vi "SmartSEM Remote API FIB mode.vi"(5 "Wait (ms)":u32, 7 "Iterations":u32=3, 8 "error in":errorcluster, 10 "FIB mode":T1(ring), 11 "ActiveX Container":refnum<k7>(container)) -> (0 "error out":errorcluster, 3 "reference out":refnum<k7>)   [LabVIEW 2018]
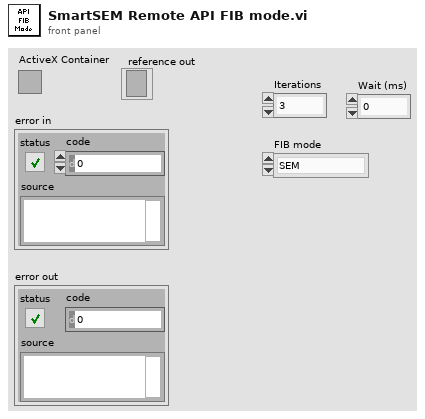
[diagram p1: front panel]
types:
  T1 = enum16{"SEM", "FIB", "Mill", "SEM + FIB", "Mill + SEM", "Drift SEM", "Drift FIB", "None", "Ext", "Ext + SEM"}
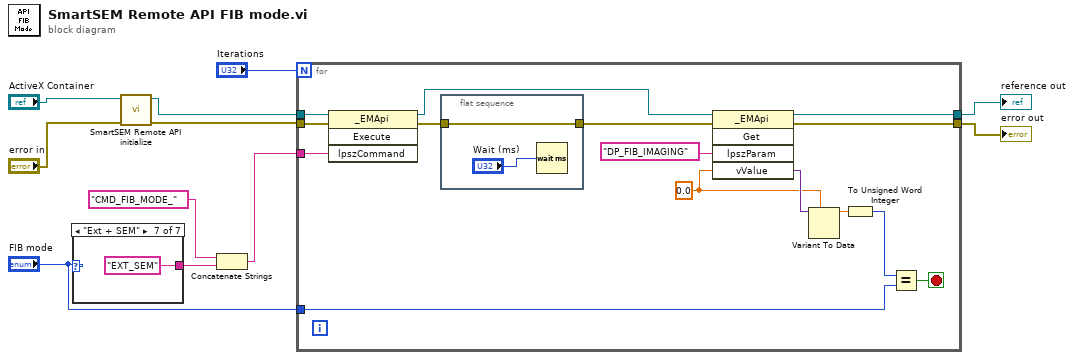
[diagram p0: block diagram]
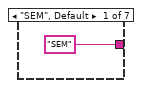
[diagram p2: hidden frame]
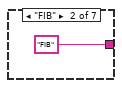
[diagram p3: hidden frame]
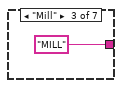
[diagram p4: hidden frame]
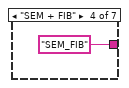
[diagram p5: hidden frame]
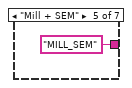
[diagram p6: hidden frame]
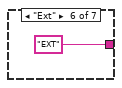
[diagram p7: hidden frame]
diagram:
  n1 = case shown="\"Ext + SEM\"" "FIB mode" {
    tunnel: ["SEM" ("lpszCommand") "FIB" ("lpszCommand") "MILL" ("lpszCommand") "SEM_FIB" ("lpszCommand") "MILL_SEM" ("lpszCommand") "EXT" ("lpszCommand") "EXT_SEM" ("lpszCommand")] -> w10
    frame "SEM", Default {
    }
    frame "FIB" {
    }
    frame "Mill" {
    }
    frame "SEM + FIB" {
    }
    frame "Mill + SEM" {
    }
    frame "Ext" {
    }
    frame "Ext + SEM" {
    }
  }
  n2 = call "SmartSEM Remote API initialize.vi"("error in"="error in", "ActiveX Container"="ActiveX Container") -> ("error out"=w1:errorcluster, "reference out"=w2:refnum<k7>)  [unwired: 8 in]
  n3 = Concatenate Strings("CMD_FIB_MODE_" ("lpszCommand"), w10) -> (w9:string)
  n4 = for {
    N: "Iterations" -> [_]
    tunnel: w2 -> [w33]
    tunnel: w9 -> [w32]
    tunnel: "FIB mode" -> [w25]
    tunnel: w1 -> [w23]
    tunnel: [w22] -> w6
    tunnel: [w21] -> w7
    stop <- w24 stop-if-true
    w28 = sgl 0.0
    n5 = invoke class="_EMApi" method="Execute"(reference=w33, error in=w23, "lpszCommand"=w32) -> (reference out=w31:refnum<k7>, error out=w20:errorcluster)  [unwired: 1 in, 2 out]
    n6 = flat-sequence {
      tunnel: [w35] -> w19
      tunnel: w20 -> [w35]
      frame #0 {
        n7 = Wait (ms)(milliseconds to wait="Wait (ms)") -> ()  [unwired: 1 out]
      }
    }
    n8 = invoke class="_EMApi" method="Get"(reference=w31, error in=w19, "lpszParam"="DP_FIB_IMAGING", "vValue"=w28) -> (reference out=w22:refnum<k7>, error out=w21:errorcluster, "vValue"=w29:variant)  [unwired: 1 in, 2 out]
    n9 = Variant To Data(type=w28, Variant=w29) -> (data=w27:sgl)  [unwired: 1 in, 1 out]
    n10 = To Unsigned Word Integer(number=w27) -> (unsigned 16bit integer=w26:u16)
    n11 = Equal?(x=w26, y=w25) -> (x = y?=w24:bool)
  }
  "error out" <- w7
  "reference out" <- w6
